vi "Generate LV Icon Text Layer.vi"(6 "Rectangle colors (black, white)":T1={"Border"=0, "Background"=16777215}, 7 "Rectangle dimension (32,32)":T2={"Width"=32, "Height"=32}, 8 "error in (no error)":errorcluster, 9 "Text settings":T3={"Font"="Small Fonts", "Alignment"=1, "Size"=8, "Center text"=TRUE, "Capitalize text"=TRUE, "Text color"={"Line 1 color"=0, "Line 2 color"=0, "Line 3 color"=0, "Line 4 color"=0}} {"Alignment" items=["left", "center", "right"]}, 10 "Text":T6, 11 "Icon in":refnum<class "Icon.lvclass">) -> (0 "error out":errorcluster, 3 "Icon out":refnum<class "Icon.lvclass">)   [LabVIEW 2020, in "LabVIEW Icon API.lvlib"]
doc: "Generating the LV Icon Text Layer requires the Text cluster.\nIn addition to the Text, it is possible to specify the visual appearance of the Text as well as a default Template Layer glyph.\n\nThe default value for the visual appearance is:\nFont: Small Fonts\nAlignment: Center\nSize: 8\nCenter text vertically: TRUE\nCapitalize text: TRUE\nColor of all four lines: Black\n\nThe default value of the Template layer is:\nSize: 32 x 32\nBorder Color: Black\nBackground Color: White"
uses:
  LabVIEW Icon API.lvlib
  lv_icon/Classes/Icon/Icon.lvclass
  lv_icon/Classes/Icon Framework/Icon Framework.lvclass
  lv_icon/Controls/Graphic.ctl
  API_Rectangle Dimension.ctl
  API_Text.ctl
  lv_icon/Controls/Alignment.ctl
  API_Text Colors.ctl
  API_Test Settings.ctl
  API_Rectangle Colors.ctl
panel:
  in  "LayerName":string="Icon Text"
  in  "Template Layer":string="Template"
  # "`"
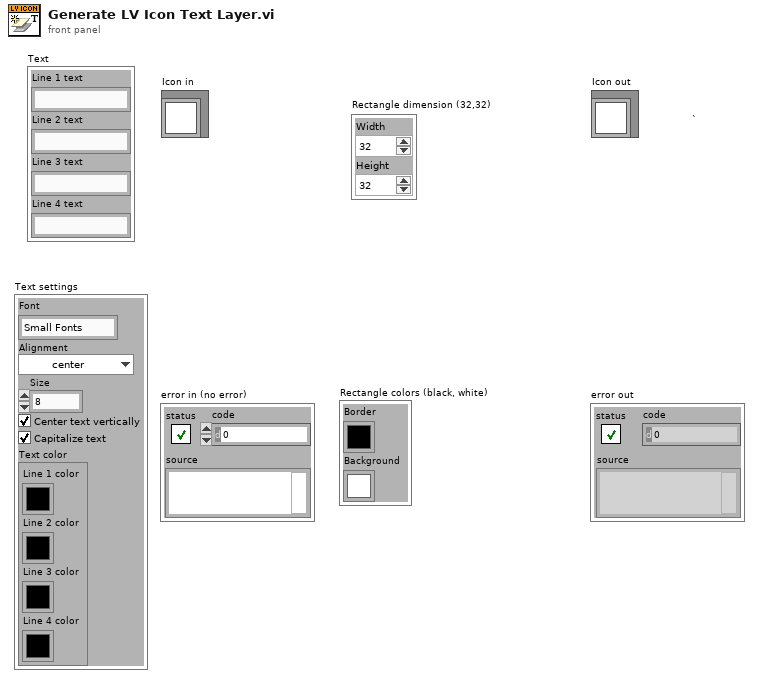
[diagram p1: front panel]
types:
  T1 = typedef "LabVIEW Icon API.lvlib/API_Rectangle Colors.ctl" = cluster{"Border":u32, "Background":u32}
  T2 = typedef "LabVIEW Icon API.lvlib/API_Rectangle Dimension.ctl" = cluster{"Width":i16, "Height":i16}
  T3 = typedef "LabVIEW Icon API.lvlib/API_Test Settings.ctl" = cluster{"Font":string, "Alignment":T4, "Size":u8, "Center text":bool, "Capitalize text":bool, "Text color":T5}
  T4 = typedef "Alignment.ctl" = u16
  T5 = typedef "LabVIEW Icon API.lvlib/API_Text Colors.ctl" = cluster{"Line 1 color":u32, "Line 2 color":u32, "Line 3 color":u32, "Line 4 color":u32}
  T6 = typedef "LabVIEW Icon API.lvlib/API_Text.ctl" = cluster{"Line 1 text":string, "Line 2 text":string, "Line 3 text":string, "Line 4 text":string}
  T7 = typedef "Graphic.ctl" = cluster{"Rectangle":cluster{"left":i16, "top":i16, "right":i16, "bottom":i16}, "Path":path, "Image":picture, "Filter":string, "FileName":string}
  T8 = typedef "BodyText.ctl" = cluster{"Line 1 text":string, "Line 2 text":string, "Line 3 text":string, "Line 4 text":string, "Line 1 color":u32, "Line 2 color":u32, "Line 3 color":u32, "Line 4 color":u32, "Body Text Spec":cluster{"Font":T9, "Alignment":T4, "Size":u8}, "Center text vertically":bool, "Capitalize Text":bool}
  T9 = typedef "Font.ctl" = string
  T10 = typedef "Layer.ctl" = cluster{"LayerIcon":picture, "LayerName":string, "Opacity":u8, "Visibility?":bool}
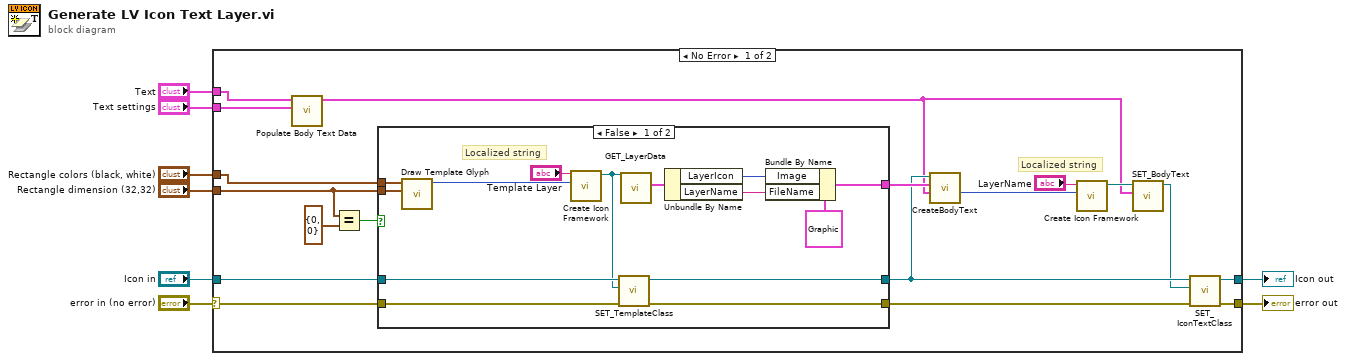
[diagram p0: block diagram]
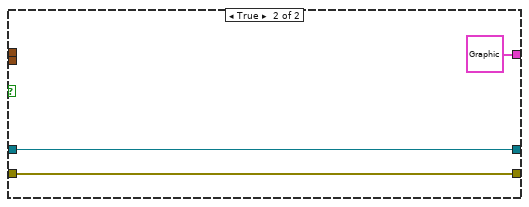
[diagram p2: hidden frame]
diagram:
  n1 = case shown="No Error" "error in (no error)" {
    selector: "error in (no error)" -> [w24 w45]
    tunnel: [w19 w45] -> w7
    tunnel: [w18 w44] -> w5
    tunnel: "Icon in" -> [w25 w44]
    tunnel: "Text" -> [w23 _]
    tunnel: "Text settings" -> [w22 _]
    tunnel: "Rectangle dimension (32,32)" -> [w10 _]
    tunnel: "Rectangle colors (black, white)" -> [w26 _]
    frame No Error {
      # "Localized string"
      n2 = call "Populate Body Text Data.vi"("Text settings"=w22, "Text"=w23) -> ("Body Text"=w13:T8)  [unwired: 9 in]
      n3 = Equal?(x=w10, y=T2 {"Width"=0, "Height"=0}) -> (x = y?=w11:bool)
      n4 = case shown="False" w11 {
        tunnel: w10 -> [w40 _]
        tunnel: w26 -> [w39 _]
        tunnel: w25 -> [w38 w43]
        tunnel: w24 -> [w37 w42]
        tunnel: [w35 T7 {"Rectangle"={"left"=0, "top"=0, "right"=0, "bottom"=0}, "Path"=path "", "Image"=bytes[0], "Filter"="", "FileName"=""} ("Path and Icon Template")] -> w21
        tunnel: [w32 w42] -> w20
        tunnel: [w31 w43] -> w17
        frame False {
          # "Localized string"
          n5 = call "Draw Template Glyph.vi"("Rectangle dimension (32,32)"=w40, "Rectangle colors (black, white)"=w39) -> ("Template Glyph"=w34:picture)  [unwired: 9 in]
          n6 = call "Create Icon Framework.vi"("Template Glyph"=w34, "Layer name"="Template Layer") -> ("Icon Framework out"=w30:refnum<class "Icon Framework.lvclass">)  [unwired: 9 in]
          n7 = call-dynamic "SET_TemplateClass.vi"("error in (no error)"=w37, "Icon Framework.lvclass"=w30, "Icon.lvclass in"=w38) -> ("error out"=w32:errorcluster, "Icon.lvclass out"=w31:refnum<class "Icon.lvclass">)  [unwired: 7 in]
          n8 = call-dynamic "GET_LayerData.vi"("Layer.lvclass in"=w30) -> ("Data"=w29:T10)  [unwired: 6 in, 4 out]
          n9 = Unbundle By Name(w29) -> ("LayerIcon"=w28:picture, "LayerName"=w27:string)
          n10 = Bundle By Name(cluster=T7 {"Rectangle"={"left"=0, "top"=0, "right"=0, "bottom"=0}, "Path"=path "", "Image"=bytes[0], "Filter"="", "FileName"=""} ("Path and Icon Template"), "Image"=w28, "FileName"=w27) -> (w35:T7)
        }
        frame True {
        }
      }
      n11 = call "CreateBodyText.vi"("Body Text"=w13, "Path and Icon Template"=w21, "Icon.lvclass in"=w17) -> ("Body Text"=w15:picture)  [unwired: 8 in]
      n12 = call "Create Icon Framework.vi"("Template Glyph"=w15, "Layer name"="LayerName") -> ("Icon Framework out"=w14:refnum<class "Icon Framework.lvclass">)  [unwired: 9 in]
      n13 = call-dynamic "SET_BodyText.vi"("Body Text"=w13, "Icon Framework.lvclass in"=w14) -> ("Icon Framework.lvclass out"=w12:refnum<class "Icon Framework.lvclass">)  [unwired: 8 in, 1 out]
      n14 = call-dynamic "SET_IconTextClass.vi"("error in (no error)"=w20, "Icon Framework.lvclass"=w12, "Icon.lvclass in"=w17) -> ("error out"=w19:errorcluster, "Icon.lvclass out"=w18:refnum<class "Icon.lvclass">)  [unwired: 7 in]
    }
    frame Error {
    }
  }
  "error out" <- w7
  "Icon out" <- w5
